vi "MHL_log_generator.vi"(8 "error in (no error)":errorcluster, 9 "Message in":string, 11 "Log in":string) -> (0 "error out":errorcluster, 3 "Message out":string)   [LabVIEW 2021]
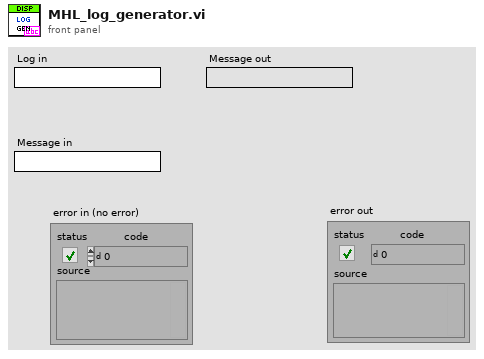
[diagram p1: front panel]
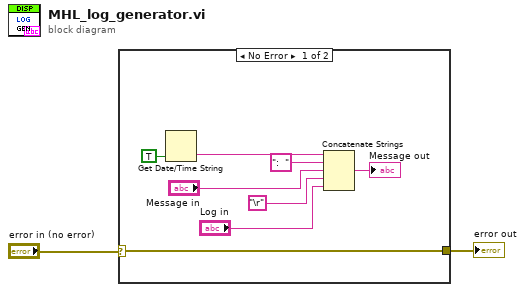
[diagram p0: block diagram]
diagram:
  n1 = case shown="No Error" "error in (no error)" {
    selector: "error in (no error)" -> [w5 w11]
    tunnel: [w5 w11] -> w1
    frame No Error {
      n2 = Get Date/Time String(want seconds? (F)=TRUE) -> (time string=w8:string)  [unwired: 2 in, 1 out]
      n3 = Concatenate Strings(w8, ":  " ("string"), "Message in", "\r", "Log in") -> (→"Message out":string)
    }
    frame Error {
    }
  }
  "error out" <- w1
